vi "testArrayToStringWithBrackets.vi"(8 "error in (no error)":errorcluster) -> (0 "error out":errorcluster)   [LabVIEW 2018]
doc: "Test the arrayToStringWithBrackets.vi"
uses:
  <vilib>/addons/_JKI Toolkits/Caraya/classes/Assert/Assert Equal Value_Variant.vi
  <vilib>/addons/_JKI Toolkits/Caraya/classes/Test/Test.lvclass
  <vilib>/addons/_JKI Toolkits/Caraya/classes/Assert/Assert.lvclass
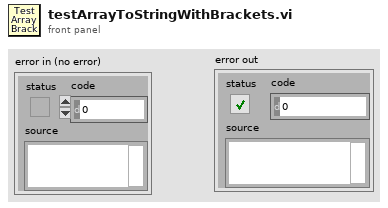
[diagram p1: front panel]
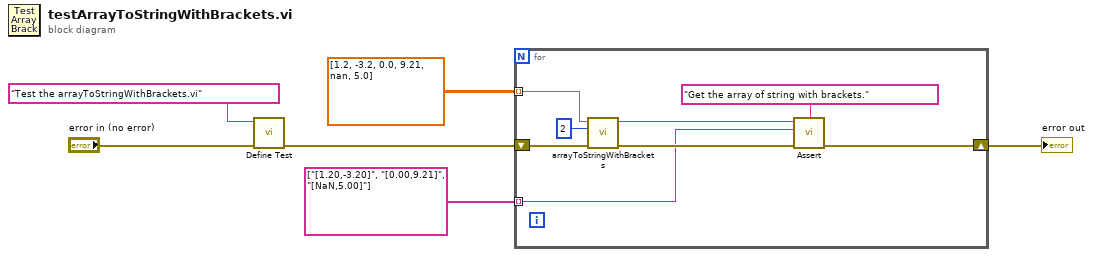
[diagram p0: block diagram]
diagram:
  n1 = call <vilib>:"Define Test.vi"("error in (no error)"="error in (no error)", "Label (VI Title)"="Test the arrayToStringWithBrackets.vi") -> ("error out"=w1:errorcluster)  [unwired: 9 in]
  n2 = for {
    tunnel: string[] ["[1.20,-3.20]", "[0.00,9.21]", "[NaN,5.00]"] ("name") -> [w11] mode=indexing
    shift-right: [w10] -> w3
    shift-left: w1 -> [w12]
    tunnel: dbl[][] [[1.2, -3.2], [0.0, 9.21], [nan, 5.0]] ("value") -> [w9] mode=indexing
    n3 = call "arrayToStringWithBrackets.vi"("presicion (0)"=u8 2, "value"=w9) -> ("String"=w8:string)  [unwired: 8 in, 1 out]
    n4 = call-poly <vilib>:"Assert.vi"("Label"="Get the array of string with brackets.", "error in (no error)"=w12, "Y"=w11, "X"=w8) -> ("error out"=w10:errorcluster)  [unwired: 7 in]
  }
  "error out" <- w3
